vi "sumData.vi"(8 "error in (no error)":errorcluster, 10 "Data Queue":refnum<queue>, 11 "Logging Configuration":T1={"Log File Base Path"=path "", "NbrIma"=1} {"NbrIma" min=1 step=1}) -> (0 "error out":errorcluster, 3 "Array":sgl[][](array[numeric]))   [LabVIEW 2020, in "Logging.lvlib"]
doc: "This VI uses the TDMS Write function to write data to a TDMS file."
uses:
  Logging Configuration.ctl
  Logging.lvlib
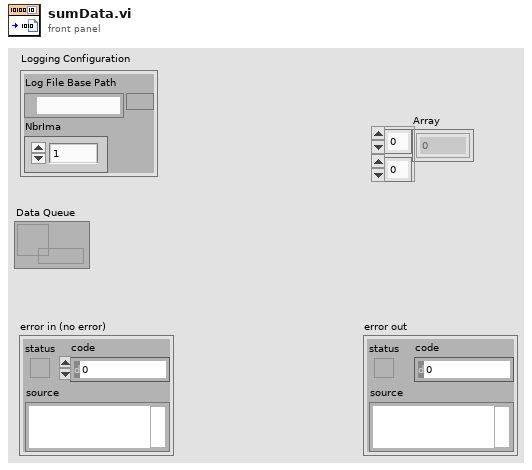
[diagram p1: front panel]
types:
  T1 = typedef "Logging.lvlib/Logging Configuration.ctl" = cluster{"Log File Base Path":path, "NbrIma":i32}
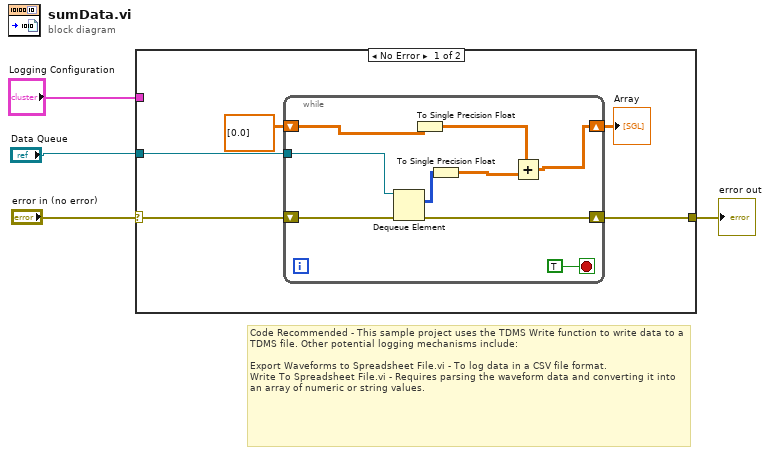
[diagram p0: block diagram]
diagram:
  # "Code Recommended - This sample project uses the TDMS Write function to write data to a TDMS file. Other potential logging mechanisms include:\n\nExport Waveforms to Spreadsheet File.vi - To log data in a CSV file format.\nWrite To Spreadsheet File.vi - Requires parsing the waveform data and converting it into an array of numeric or string values."
  n1 = case shown="No Error" "error in (no error)" {
    selector: "error in (no error)" -> [w6 w19]
    tunnel: "Logging Configuration" -> [_ _]
    tunnel: "Data Queue" -> [w7 _]
    tunnel: [w9 w19] -> w3
    frame No Error {
      n2 = while {
        tunnel: w7 -> [w17]
        shift-right: [w16] -> w9
        shift-left: w6 -> [w18]
        shift-right: [w14] -> w8
        shift-left: sgl[][] [[0.0]] -> [w15]
        stop <- TRUE stop-if-true
        n3 = Dequeue Element(queue=w17, error in (no error)=w18) -> (element=w12:u16[][], error out=w16:errorcluster)  [unwired: 1 in, 2 out]
        n4 = To Single Precision Float(number=w15) -> (single precision float=w10:sgl[][])
        n5 = To Single Precision Float(number=w12) -> (single precision float=w11:sgl[][])
        n6 = Add(x=w10, y=w11) -> (x+y=w14:sgl[][])
      }
      "Array" <- w8
    }
    frame Error {
    }
  }
  "error out" <- w3
